vi "Close Instrument.vi"(8 "error in (no error)":errorcluster, 11 "instrument.PPMS":refnum<class "instrument.PPMS.lvclass">) -> (0 "error out":errorcluster, 3 "instrument.PPMS out":refnum<class "instrument.PPMS.lvclass">)   [LabVIEW 2019, in "instrument.PPMS.lvclass"]
uses:
  instrument.PPMS.lvclass
  instrument.PPMS.lvclass/instrument.PPMS.ctl
  C:/Users/patrick/Documents/GitHub/PPMS-Monitor-and-Control/lvsrc/drivers/QDInstrument_LabView/QDInstrument.dll
  drivers/QDInstrument_LabView/QDInstrument.dll
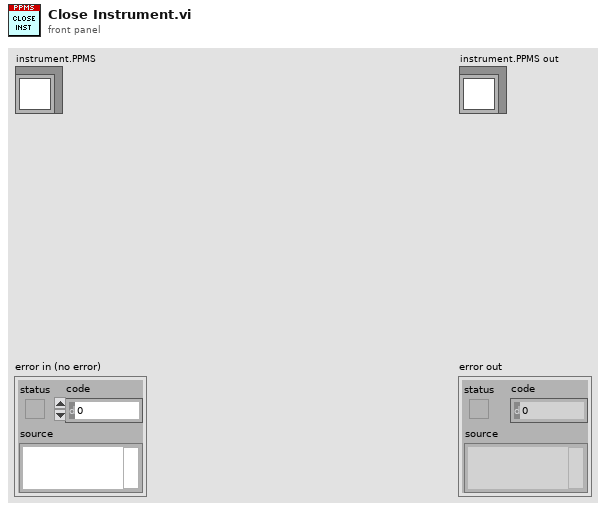
[diagram p1: front panel]
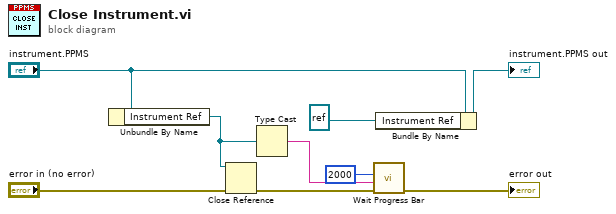
[diagram p0: block diagram]
diagram:
  n1 = Unbundle By Name("instrument.PPMS") -> ("Instrument Ref"=w2:refnum<k24>)
  n2 = Close Reference(reference=w2, error in (no error)="error in (no error)") -> (error out=w4:errorcluster)
  n3 = Type Cast(x=w2) -> (*(type *) &x=w1:string)  [unwired: 1 in]
  n4 = call "Wait Progress Bar.vi"("error in (no error)"=w4, "Message [Shutting Down...]"=w1, "wait (ms)"=u32 2000 ("milliseconds to wait")) -> ("error out"=→"error out":errorcluster)  [unwired: 8 in]
  n5 = Bundle By Name(cluster="instrument.PPMS", "Instrument Ref"=refnum<k24> refnum) -> (→"instrument.PPMS out":refnum<class "instrument.PPMS.lvclass">)
